vi "Disabled channel logic 2ch.vi"(7 "reset":bool, 9 "input valid":bool, 10 "U32 data in":u32[](array[numeric])=[0, 0], 11 "enabled channels":u32) -> (1 "data ready":bool, 2 "U32 data out":u32[](array[numeric]))   [LabVIEW 2025, in "niUSRP Stream Control (DMA) v1 FPGA.lvclass"]
uses:
  niUSRP Stream Control (DMA) v1 FPGA.lvclass
  niUSRP Stream Control (DMA) v1 FPGA.lvclass/niUSRP Stream Control (DMA) v1 FPGA.ctl
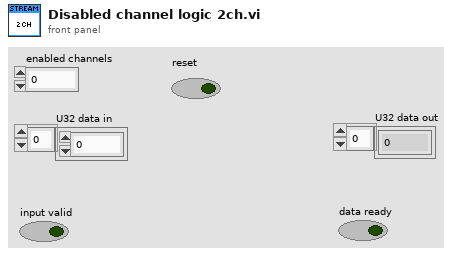
[diagram p1: front panel]
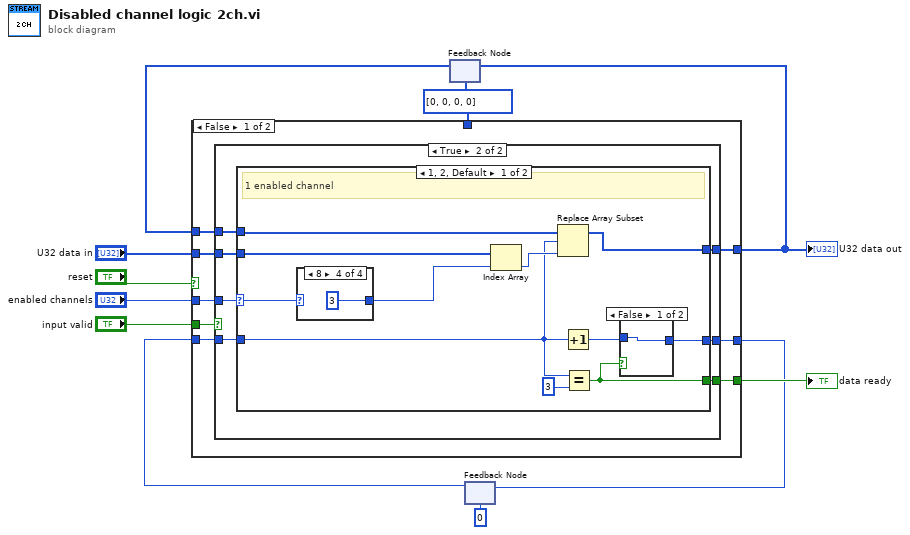
[diagram p0: block diagram]
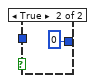
[diagram p3: hidden frame]
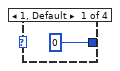
[diagram p4: hidden frame]
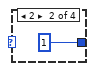
[diagram p5: hidden frame]
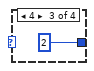
[diagram p6: hidden frame]
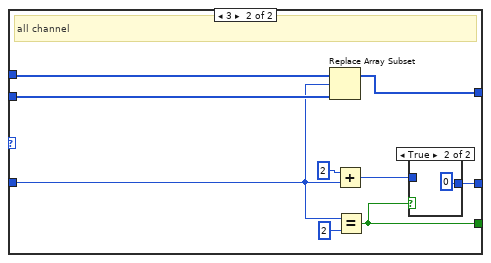
[diagram p7: hidden frame]
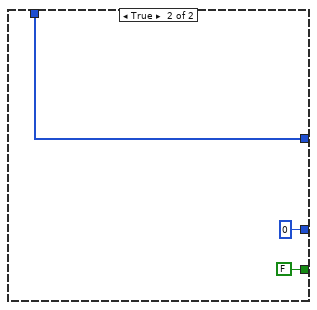
[diagram p9: hidden frame]
diagram:
  w1 = u32[] [0, 0, 0, 0]
  n1 = feedback #1(w1) -> (w11:u32[])
  n2 = feedback #2(u8 0) -> (w5:u8)
  n3 = case shown="False" "reset" {
    tunnel: w11 -> [w19 _]
    tunnel: "input valid" -> [w18 _]
    tunnel: "U32 data in" -> [w17 _]
    tunnel: [w16 w58] -> w8
    tunnel: "enabled channels" -> [w15 _]
    tunnel: w5 -> [w14 _]
    tunnel: [w13 FALSE] -> w4
    tunnel: [w12 u8 0] -> w3
    tunnel: w1 -> [_ w58]
    frame False {
      n4 = case shown="True" w18 {
        selector: w18 -> [w22 _]
        tunnel: w19 -> [w20 w29]
        tunnel: w15 -> [_ w28]
        tunnel: w17 -> [_ w27]
        tunnel: w14 -> [w21 w26]
        tunnel: [w20 w25] -> w16
        tunnel: [w21 w24] -> w12
        tunnel: [w22 w23] -> w13
        frame False {
        }
        frame True {
          n5 = case shown="1, 2, Default" w28 {
            selector: w28 -> [w39 _]
            tunnel: w27 -> [w35 w51]
            tunnel: [w38 w53] -> w25
            tunnel: [w31 w49] -> w23
            tunnel: w26 -> [w33 w50]
            tunnel: [w30 w48] -> w24
            tunnel: w29 -> [w37 w54]
            frame 1, 2, Default {
              # "1 enabled channel"
              n6 = case shown="8" w39 {
                tunnel: [0 ("index") 1 ("index") 2 ("index") 3 ("index")] -> w34
                frame 1, Default {
                }
                frame 2 {
                }
                frame 4 {
                }
                frame 8 {
                }
              }
              n7 = Index Array(array=w35, index=w34) -> (element=w36:u32)
              n8 = Replace Array Subset(array=w37, new element=w36, index=w33) -> (w38:u32[])
              n9 = Increment(x=w33) -> (x+1=w32:u8)
              n10 = Equal?(x=w33, y=u8 3) -> (x = y?=w31:bool)
              n11 = case shown="False" w31 {
                tunnel: [w41 u8 0] -> w30
                tunnel: w32 -> [w41 _]
                frame False {
                }
                frame True {
                }
              }
            }
            frame 3 {
              # "all channel"
              n12 = Replace Array Subset(array=w54, new element=w51, index=w50) -> (w53:u32[])
              n13 = Add(x=u8 2, y=w50) -> (x+y=w47:u8)
              n14 = Equal?(x=w50, y=u8 2) -> (x = y?=w49:bool)
              n15 = case shown="True" w49 {
                tunnel: [w56 u8 0] -> w48
                tunnel: w47 -> [w56 _]
                frame False {
                }
                frame True {
                }
              }
            }
          }
        }
      }
    }
    frame True {
    }
  }
  "data ready" <- w4
  "U32 data out" <- w8
  n16 = feedback-in #1(w8) -> ()
  n17 = feedback-in #2(w3) -> ()
